vi "Export Custom Device.vi"(8 "error in":errorcluster, 10 "path":path, 11 "custom device ref in":T1 format="%.0x") -> (0 "error out":errorcluster, 3 "custom device ref out":T1 format="%.0x")   [LabVIEW 2020, in "AIM ARINC 429 Scripting.lvlib"]
uses:
  AIM ARINC 429 Scripting.lvlib
  <vilib>/NI/VeriStand Custom Device Serialization/Custom Device Serialization.lvlib
  <vilib>/NI VeriStand/Custom Device API/Custom Device Item Ref.ctl
  <vilib>/NI VeriStand/Custom Device API/Custom Device API.lvlib
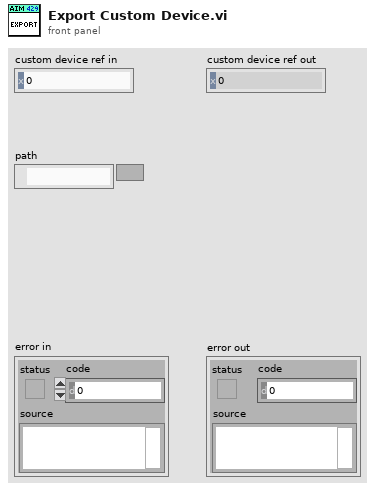
[diagram p1: front panel]
types:
  T1 = typedef "Custom Device API.lvlib/Custom Device Item Ref.ctl" = u64
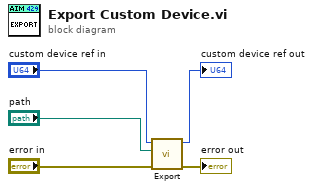
[diagram p0: block diagram]
diagram:
  n1 = call <vilib>:"Export.vi"("error in"="error in", "path"="path", "item in"="custom device ref in") -> ("error out"=→"error out":errorcluster, "item out"=→"custom device ref out":T1)  [unwired: 7 in]
